vi "Actor Core.vi"(8 "error in":errorcluster, 11 "UI in":refnum<class "UI.lvclass">) -> (0 "error out":errorcluster, 3 "Actor out":refnum<class "Actor.lvclass">)   [LabVIEW 2015, in "UI.lvlib" / "UI.lvclass"]
doc: "(<B>Filename</B>: Actor Framework.lvlib:Actor.lvclass:Actor Core.vi)\n\nReceives messages to the actor, reacts to them, and initiates any error handling that may shut the actor down.\n\nDescendant classes may override this VI to append parallel tasks for the actor to complete while it handles messages. Overrides use the Call Parent Method node."
uses:
  UI.lvclass
  <vilib>/ActorFramework/Actor/Actor.lvclass
  Sequencer/Sequencer/Sequencer.lvclass
  <vilib>/ActorFramework/Stop Msg/Stop Msg.lvclass
  Ctl Refs.ctl
  UI Messages/Update Refs Msg/Update Refs Msg.lvclass
  UI Messages/Add Channel to Sequence Msg/Add Channel to Sequence Msg.lvclass
  UI Messages/Remove Channels from Sequence Msg/Remove Channels from Sequence Msg.lvclass
  Sequencer/Sequencer Messages/Open Channel Panel Msg/Open Channel Panel Msg.lvclass
  Sequencer/SequencerInfo.lvclass
  Sequencer/SequencerConfig.lvclass
  Sequencer/Sequencer Messages/Broadcast SequencerInfo Msg/Broadcast SequencerInfo Msg.lvclass
  Sequencer/Sequencer Messages/Play Sequence Msg/Play Sequence Msg.lvclass
  <vilib>/MGI/Monitored Actor/Monitored Actor/Monitored Actor/Monitored Actor.lvclass
  Simulated Sequencer/Simulated Sequencer/Simulated Sequencer.lvclass
  DAQmx Sequencer/DAQmx Sequencer/DAQmx Sequencer.lvclass
  Sequencer/Sequencer/ChannelTypes.ctl
panel:
  in  "Play Sequence":bool
  in  "Boolean":bool
  in  "Display Channel":bool
  in  "Delete Channels":bool
  in  "Used Channels":i32(listbox)
  in  "Stop Program":bool
  in  "Add Channel":bool
  in  "Type":T1
  in  "Channel":u16(ring)
  in  "Basic Params":cluster{"Sample Rate":dbl, "Buffer Size":dbl}
  in  "Device":u16(ring)
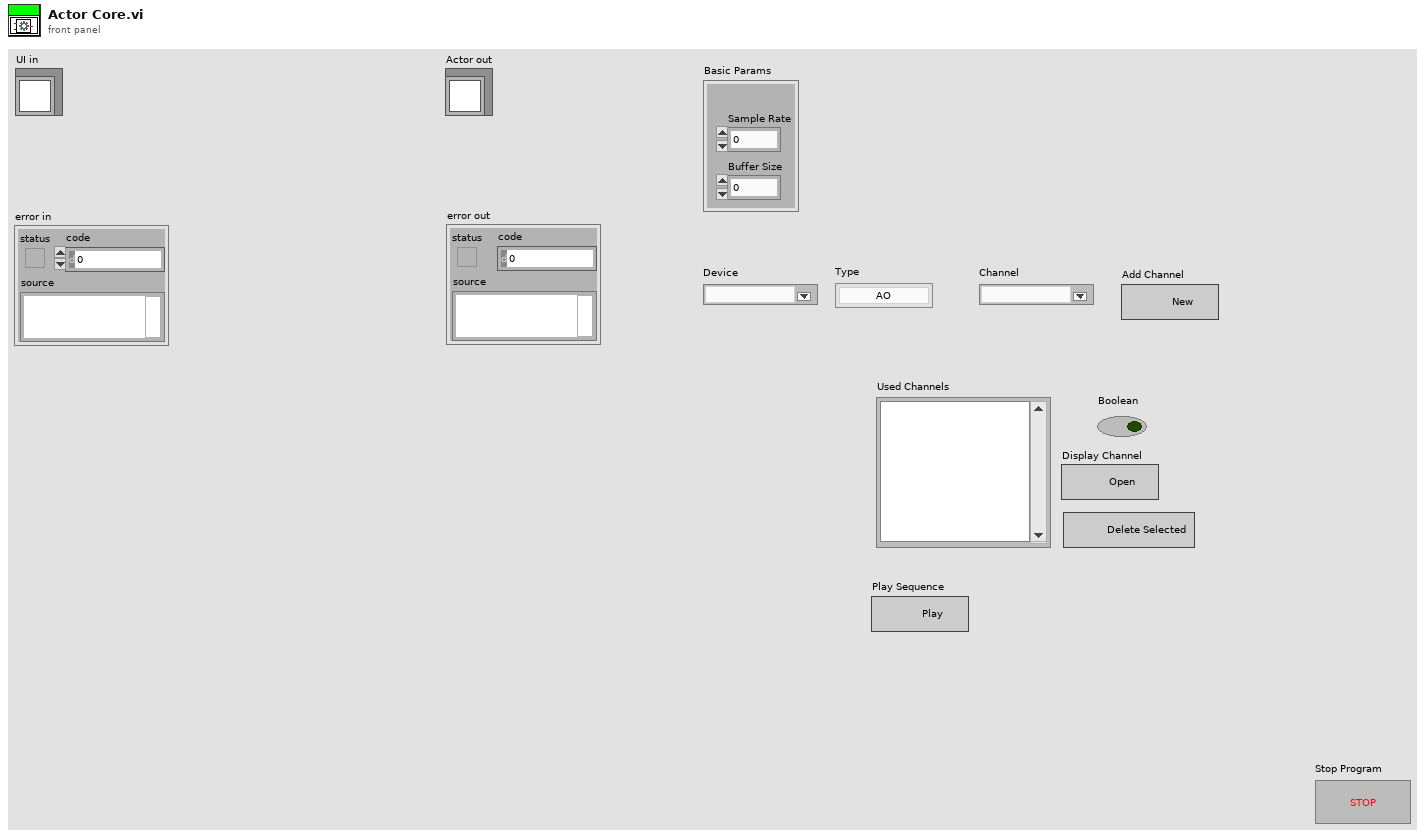
[diagram p1: front panel]
types:
  T1 = typedef "Sequencer.lvlib/Sequencer.lvclass/ChannelTypes.ctl" = enum16{"AO", "DO", "AI"}
  T2 = typedef "UI.lvlib/UI.lvclass/Ctl Refs.ctl" = cluster{"Basic Params":refnum<vi>, "Type":refnum<vi>, "Channel":refnum<vi>, "Device":refnum<vi>, "Used Channels":refnum<vi>, "Add Channel":refnum<vi>, "Stop Program":refnum<vi>, "Delete Channels":refnum<vi>, "Display Channel":refnum<vi>, "Play Sequence":refnum<vi>}
  T3 = enum8{"Enabled", "Disabled", "Disabled and Grayed Out"}
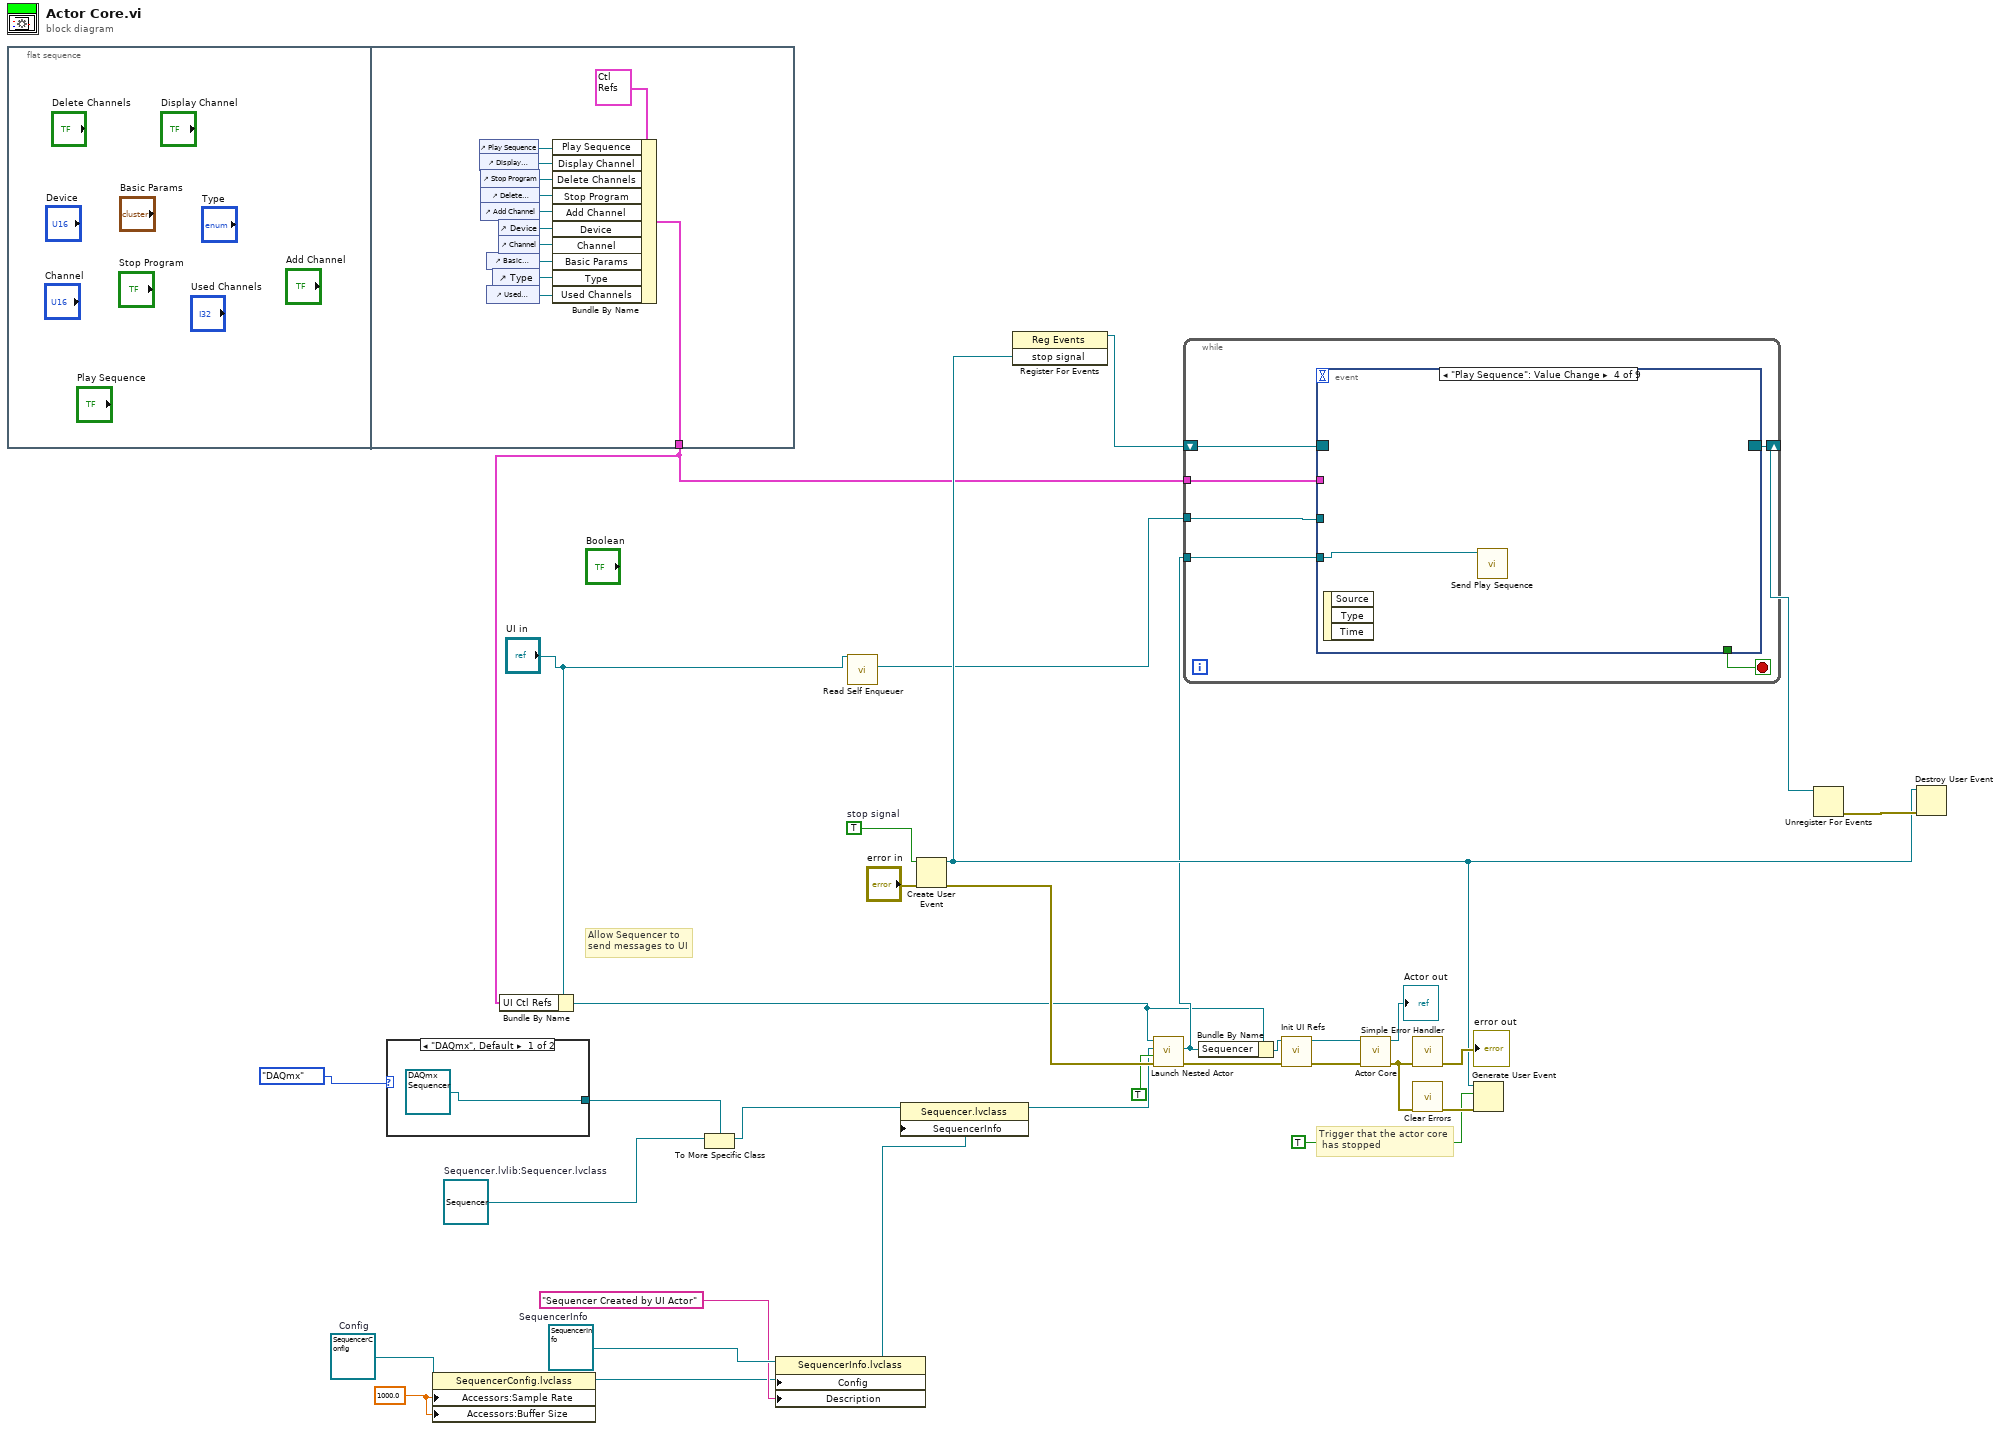
[diagram p0: block diagram]
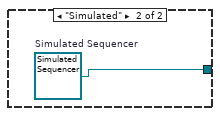
[diagram p2: hidden frame]
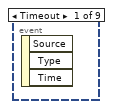
[diagram p3: hidden frame]
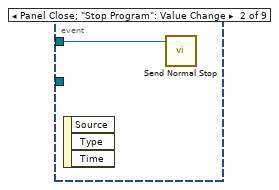
[diagram p4: hidden frame]
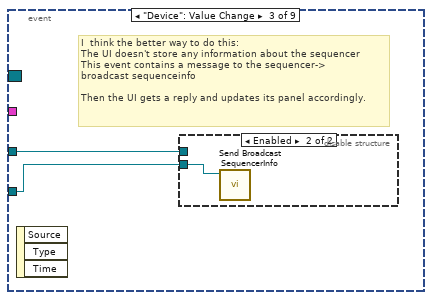
[diagram p5: hidden frame]
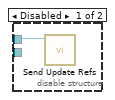
[diagram p6: hidden frame]
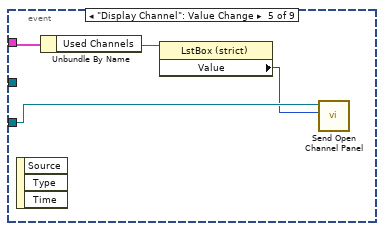
[diagram p7: hidden frame]
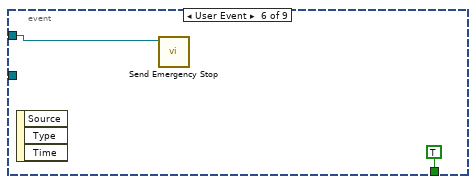
[diagram p8: hidden frame]
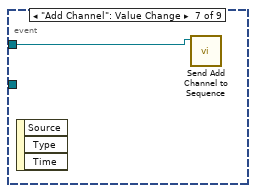
[diagram p9: hidden frame]
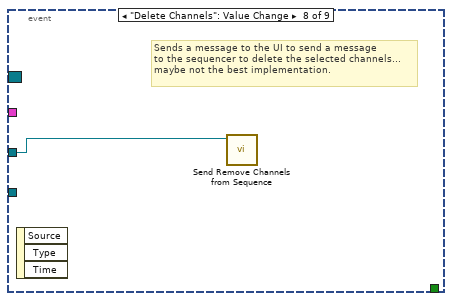
[diagram p10: hidden frame]
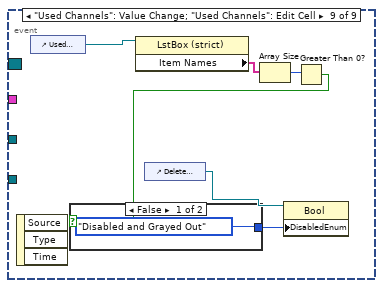
[diagram p11: hidden frame]
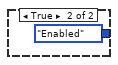
[diagram p12: hidden frame]
diagram:
  w5 = 1000.0 ("Sample Rate")
  w7 = refnum<class "SequencerConfig.lvclass"> refnum  # Config
  w10 = refnum<class "SequencerInfo.lvclass"> refnum  # SequencerInfo
  w32 = TRUE  # stop signal
  w3 = refnum<class "Sequencer.lvclass"> refnum  # Sequencer.lvlib:Sequencer.lvclass
  # "Allow Sequencer to\nsend messages to UI"
  # "Trigger that the actor core\n has stopped"
  n1 = flat-sequence {
    tunnel: [w44] -> w12
    frame #0 {
    }
    frame #1 {
      n2 = control-ref of="Play Sequence"() -> (w34:refnum<vi>)
      n3 = control-ref of="Display Channel"() -> (w35:refnum<vi>)
      n4 = control-ref of="Stop Program"() -> (w37:refnum<vi>)
      n5 = control-ref of="Delete Channels"() -> (w36:refnum<vi>)
      n6 = control-ref of="Add Channel"() -> (w38:refnum<vi>)
      n7 = control-ref of="Basic Params"() -> (w43:refnum<vi>)
      n8 = control-ref of="Used Channels"() -> (w39:refnum<vi>)
      n9 = control-ref of="Type"() -> (w42:refnum<vi>)
      n10 = control-ref of="Device"() -> (w40:refnum<vi>)
      n11 = control-ref of="Channel"() -> (w41:refnum<vi>)
      n12 = Bundle By Name(cluster=T2 {"Basic Params"=refnum, "Type"=refnum, "Channel"=refnum, "Device"=refnum, "Used Channels"=refnum, "Add Channel"=refnum, "Stop Program"=refnum, "Delete Channels"=refnum, "Display Channel"=refnum, "Play Sequence"=refnum} ("output cluster"), "Play Sequence"=w34, "Display Channel"=w35, "Delete Channels"=w36, "Stop Program"=w37, "Add Channel"=w38, "Device"=w40, "Channel"=w41, "Basic Params"=w43, "Type"=w42, "Used Channels"=w39) -> (w44:T2)
    }
  }
  n13 = case shown="\"DAQmx\", Default" enum16{"DAQmx", "Simulated"}."DAQmx" ("Enum") {
    tunnel: [refnum<class "DAQmx Sequencer.lvclass"> refnum ("DAQmx Sequencer.lvlib:DAQmx Sequencer.lvclass") w47] -> w1
    frame "DAQmx", Default {
    }
    frame "Simulated" {
      w47 = refnum<class "Simulated Sequencer.lvclass"> refnum  # Simulated Sequencer
    }
  }
  n14 = property class="SequencerConfig.lvclass"(reference=w7, "Accessors:Sample Rate"=w5, "Accessors:Buffer Size"=w5) -> (reference out=w6:refnum<class "SequencerConfig.lvclass">)  [unwired: 1 in, 1 out]
  n15 = Bundle By Name(cluster="UI in", "UI Ctl Refs"=w12) -> (w17:refnum<class "UI.lvclass">)
  n16 = To More Specific Class(target class=w1, reference=w3) -> (specific class reference=w4:refnum<class "Sequencer.lvclass">)  [unwired: 1 in, 1 out]
  n17 = property class="SequencerInfo.lvclass"(reference=w10, "Config"=w6, "Description"="Sequencer Created by UI Actor") -> (reference out=w9:refnum<class "SequencerInfo.lvclass">)  [unwired: 1 in, 1 out]
  n18 = call <vilib>:"Read Self Enqueuer.vi"("Actor"="UI in") -> ("Self Enqueuer"=w19:refnum<class "Message Enqueuer.lvclass">)  [unwired: 10 in]
  n19 = property class="Sequencer.lvclass"(reference=w4, "SequencerInfo"=w9) -> (reference out=w11:refnum<class "Sequencer.lvclass">)  [unwired: 1 in, 1 out]
  n20 = Create User Event(user event datatype=w32, error in="error in") -> (user event=w23:refnum<user-event>, error out=w24:errorcluster)
  n21 = register-events(w23) -> (reference out=w28:refnum<event-registration>)  [unwired: 2 in, 1 out]
  n22 = call <vilib>:"Launch Nested Actor.vi"("error in (no error)"=w24, "Auto-stop? (T)"=TRUE, "Nested Actor"=w11, "Caller Actor in"=w17) -> ("error out"=w14:errorcluster, "Nested Actor's Enqueuer"=w20:refnum<class "Message Enqueuer.lvclass">)  [unwired: 5 in, 1 out]
  n23 = while {
    tunnel: w19 -> [w53]
    tunnel: w20 -> [w52]
    shift-right: [w49] -> w26
    shift-left: w28 -> [w50]
    tunnel: w12 -> [w48]
    stop <- w51 stop-if-true
    n24 = event shown="[3] \"Play Sequence\": Value Change" {
      selector: w50 -> [_ _ _ _ _ _ _ _ _]
      dyn-events: [_ _ _ _ _ _ _ _ _] -> w49
      timeout: _ -> [_ _ _ _ _ _ _ _ _]
      tunnel: w53 -> [_ w54 w56 _ _ w65 w66 w67 _]
      tunnel: w52 -> [_ _ w55 w59 w63 _ _ _ _]
      tunnel: [_ _ _ _ _ TRUE _ _ _] -> w51
      tunnel: w48 -> [_ _ _ _ w62 _ _ _ _]
      event Timeout {
        n25 = event-data() -> ()  [unwired: 1 in, 3 out]
      }
      event Panel Close; "Stop Program": Value Change {
        n26 = event-data() -> ()  [unwired: 1 in, 3 out]
        n27 = call <vilib>:"Send Normal Stop.vi"("Message Enqueuer"=w54) -> ()  [unwired: 10 in, 1 out]
      }
      event "Device": Value Change {
        # "I  think the better way to do this:\nThe UI doesn't store any information about the sequencer\nThis event contains a message to the sequencer-> \nbroadcast sequenceinfo\n\nThen the UI gets a reply and updates its panel accordingly."
        n28 = event-data() -> ()  [unwired: 1 in, 3 out]
        n29 = disable-structure shown="Enabled" {
          disable-tunnel: w56 -> [w57 _]
          disable-tunnel: w55 -> [_ w58]
          frame Disabled {
            n30 = call "Send Update Refs.vi"("Message Enqueuer in"=w57) -> ()  [unwired: 9 in, 2 out]
          }
          frame Enabled {
            n31 = call "Send Broadcast SequencerInfo.vi"("Message Enqueuer in"=w58) -> ()  [unwired: 9 in, 2 out]
          }
        }
      }
      event "Play Sequence": Value Change {
        n32 = event-data() -> ()  [unwired: 1 in, 3 out]
        n33 = call "Send Play Sequence.vi"("Message Enqueuer in"=w59) -> ()  [unwired: 9 in, 2 out]
      }
      event "Display Channel": Value Change {
        n34 = event-data() -> ()  [unwired: 1 in, 3 out]
        n35 = Unbundle By Name(w62) -> ("Used Channels"=w61:refnum<vi>)
        n36 = property class="LstBox (strict)"(reference=w61) -> ("Value"=w60:i32)  [unwired: 1 in, 2 out]
        n37 = call "Send Open Channel Panel.vi"("Channel Index"=w60, "Message Enqueuer in"=w63) -> ()  [unwired: 8 in, 2 out]
      }
      event User Event {
        n38 = event-data() -> ()  [unwired: 1 in, 3 out]
        n39 = call <vilib>:"Send Emergency Stop.vi"("Message Enqueuer"=w65) -> ()  [unwired: 10 in, 1 out]
      }
      event "Add Channel": Value Change {
        n40 = event-data() -> ()  [unwired: 1 in, 3 out]
        n41 = call "Send Add Channel to Sequence.vi"("Message Enqueuer in"=w66) -> ()  [unwired: 9 in, 2 out]
      }
      event "Delete Channels": Value Change {
        # "Sends a message to the UI to send a message\nto the sequencer to delete the selected channels...\nmaybe not the best implementation."
        n42 = event-data() -> ()  [unwired: 1 in, 3 out]
        n43 = call "Send Remove Channels from Sequence.vi"("Message Enqueuer in"=w67) -> ()  [unwired: 9 in, 2 out]
      }
      event "Used Channels": Value Change; "Used Channels": Edit Cell {
        n44 = event-data() -> ()  [unwired: 1 in, 3 out]
        n45 = control-ref of="Used Channels"() -> (w71:refnum<vi>)
        n46 = property class="LstBox (strict)"(reference=w71) -> ("Item Names"=w70:string[])  [unwired: 1 in, 2 out]
        n47 = control-ref of="Delete Channels"() -> (w72:refnum<vi>)
        n48 = Array Size(array=w70) -> (size(s)=w69:i32)
        n49 = Greater Than 0?(x=w69) -> (x > 0?=w68:bool)
        n50 = case shown="False" w68 {
          tunnel: [T3."Disabled and Grayed Out" ("Disabled") T3."Enabled" ("Disabled")] -> w73
          frame False {
          }
          frame True {
          }
        }
        n51 = property class="Bool"(reference=w72, "DisabledEnum"=w73) -> ()  [unwired: 1 in, 2 out]
      }
    }
  }
  n52 = Bundle By Name(cluster=w17, "Sequencer"=w20) -> (w16:refnum<class "UI.lvclass">)
  n53 = call "Init UI Refs.vi"("error in (no error)"=w14, "UI in"=w16) -> ("error out"=w13:errorcluster, "UI out"=w15:refnum<class "UI.lvclass">)  [unwired: 8 in]
  n54 = call-parent "Actor Core.vi"("error in"=w13, "Actor in"=w15) -> ("error out"=w30:errorcluster, "Actor out"=→"Actor out":refnum<class "Actor.lvclass">)  [unwired: 8 in]
  n55 = call <vilib>:"Simple Error Handler.vi"("error in (no error)"=w30) -> ("error out"=→"error out":errorcluster)  [unwired: 4 in, 4 out]
  n56 = call <vilib>:"Clear Errors.vi"("error in (no error)"=w30) -> ("error out"=w29:errorcluster)  [unwired: 5 in, 1 out]
  n57 = Generate User Event(user event=w23, event data cluster=TRUE ("event data"), error in=w29) -> ()  [unwired: 1 in, 2 out]
  n58 = Unregister For Events(event registration refnum=w26) -> (error out=w27:errorcluster)  [unwired: 1 in]
  n59 = Destroy User Event(user event=w23, error in=w27) -> ()  [unwired: 1 out]
